vi "WF0_RLE.vi"(0 "connection ID in":refnum<k5>, 1 "TxPulseRleA":string, 2 "Mode control":enum32{"D-mode", "B-mode"}(ring), 3 "Timeout (ms)":i32=40000000, 4 "TxFrequencyIndex":i8) -> (5 "connection ID out":refnum<k5>, 7 "Timeout (ms) out":i32)   [LabVIEW 2016]
uses:
  TemperatureMeasure/Thermal_type.vi
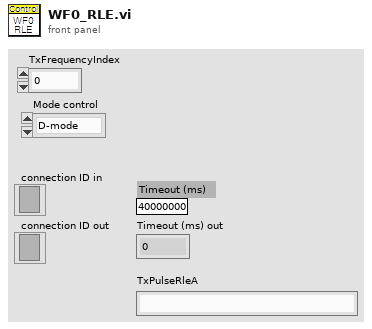
[diagram p1: front panel]
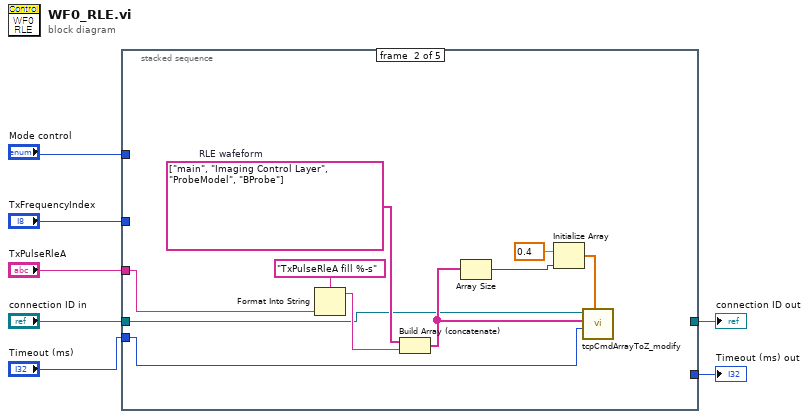
[diagram p0: block diagram]
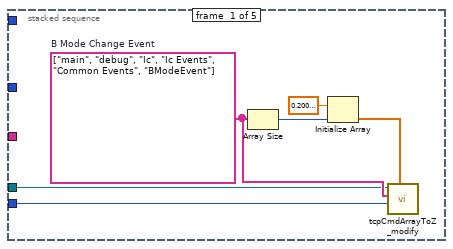
[diagram p2: hidden frame]
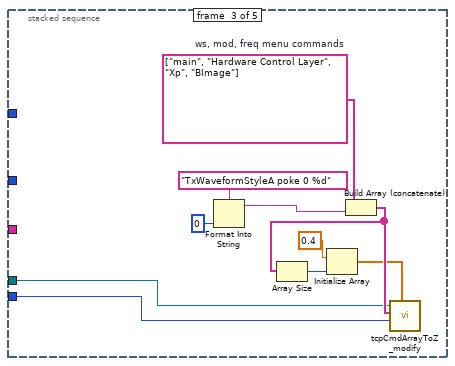
[diagram p3: hidden frame]
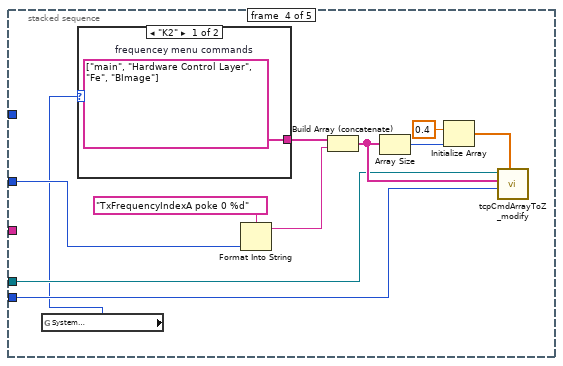
[diagram p4: hidden frame]
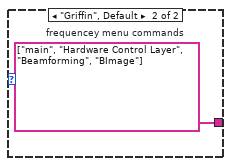
[diagram p5: hidden frame]
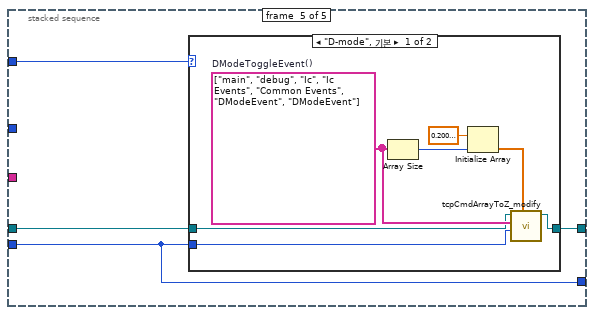
[diagram p6: hidden frame]
diagram:
  n1 = stacked-sequence {
    tunnel: "connection ID in" -> [w9 w15 w26 w36 w48]
    tunnel: "Timeout (ms)" -> [w8 w14 w25 w37 w49]
    tunnel: [_ _ _ _ w50] -> w5
    tunnel: [_ _ _ _ w49] -> w4
    tunnel: "TxPulseRleA" -> [_ w16 _ _ _]
    tunnel: "Mode control" -> [_ _ _ _ w47]
    tunnel: "TxFrequencyIndex" -> [_ _ _ w35 _]
    frame #0 {
      w13 = string[] ["main", "debug", "Ic", "Ic Events", "Common Events", "BModeEvent"]  # B Mode Change Event
      n2 = Array Size(array=w13) -> (size(s)=w10:i32)
      n3 = Initialize Array(sgl 0.2 ("element"), w10) -> (w12:sgl[])
      n4 = call "tcpCmdArrayToZ_modify.vi"("Delay (sec)"=w12, "Timeout (ms)"=w8, "Command array"=w13, "connection ID in"=w9) -> ()  [unwired: 3 in, 5 out]
    }
    frame #1 {
      w17 = string[] ["main", "Imaging Control Layer", "ProbeModel", "BProbe"]  # RLE wafeform
      n5 = Format Into String(format string="TxPulseRleA fill %-s" ("Format String"), w16) -> (resulting string=w21:string)  [unwired: 2 in, 1 out]
      n6 = Build Array (concatenate)(w17, w21) -> (w22:string[])
      n7 = Array Size(array=w22) -> (size(s)=w23:i32)
      n8 = Initialize Array(0.4 ("element"), w23) -> (w19:dbl[])
      n9 = call "tcpCmdArrayToZ_modify.vi"("Delay (sec)"=w19, "Timeout (ms)"=w14, "Command array"=w22, "connection ID in"=w15) -> ()  [unwired: 3 in, 5 out]
    }
    frame #2 {
      w32 = string[] ["main", "Hardware Control Layer", "Xp", "BImage"]  # ws, mod, freq menu commands
      n10 = Format Into String(format string="TxWaveformStyleA poke 0 %d" ("Format String"), i8 0 ("입력 1")) -> (resulting string=w31:string)  [unwired: 2 in, 1 out]
      n11 = Build Array (concatenate)(w32, w31) -> (w30:string[])
      n12 = Array Size(array=w30) -> (size(s)=w29:i32)
      n13 = Initialize Array(0.4 ("원소"), w29) -> (w27:dbl[])
      n14 = call "tcpCmdArrayToZ_modify.vi"("Delay (sec)"=w27, "Timeout (ms)"=w25, "Command array"=w30, "connection ID in"=w26) -> ()  [unwired: 3 in, 5 out]
    }
    frame #3 {
      n15 = global read "Thermal_type.vi" "System \nSelection"() -> (w34:enum32{"Common", "Frosk", "Griffin", "K2"})
      n16 = case shown="\"K2\"" w34 {
        tunnel: [w45 w46] -> w40
        frame "K2" {
          w45 = string[] ["main", "Hardware Control Layer", "Fe", "BImage"]  # frequencey menu commands
        }
        frame "Griffin", Default {
          w46 = string[] ["main", "Hardware Control Layer", "Beamforming", "BImage"]  # frequencey menu commands
        }
      }
      n17 = Format Into String(format string="TxFrequencyIndexA poke 0 %d" ("초기 문자열"), w35) -> (resulting string=w41:string)  [unwired: 2 in, 1 out]
      n18 = Build Array (concatenate)(w40, w41) -> (w38:string[])
      n19 = Array Size(array=w38) -> (size(s)=w43:i32)
      n20 = Initialize Array(0.4 ("원소"), w43) -> (w42:dbl[])
      n21 = call "tcpCmdArrayToZ_modify.vi"("Delay (sec)"=w42, "Timeout (ms)"=w37, "Command array"=w38, "connection ID in"=w36) -> ()  [unwired: 3 in, 5 out]
    }
    frame #4 {
      n22 = case shown="\"D-mode\", 기본" w47 {
        tunnel: [w53 w58] -> w50
        tunnel: w49 -> [w52 _]
        tunnel: w48 -> [w51 w58]
        frame "D-mode", Default {
          w54 = string[] ["main", "debug", "Ic", "Ic Events", "Common Events", "DModeEvent", "DModeEvent"]  # DModeToggleEvent()
          n23 = Array Size(array=w54) -> (size(s)=w57:i32)
          n24 = Initialize Array(sgl 0.2 ("element"), w57) -> (w55:sgl[])
          n25 = call "tcpCmdArrayToZ_modify.vi"("Delay (sec)"=w55, "Timeout (ms)"=w52, "Command array"=w54, "connection ID in"=w51) -> ("connection ID out"=w53:refnum<k5>)  [unwired: 3 in, 4 out]
        }
        frame "B-mode" {
        }
      }
    }
  }
  "connection ID out" <- w5
  "Timeout (ms) out" <- w4
